vi "Begin_Turret.vi"() -> (0 "error out":errorcluster)   [LabVIEW 2012]
uses:
  <vilib>/Rock Robotics/WPI/CAN/Jaguar/SubVIs/WPI_CANJaguar_ControlMode.ctl
  <vilib>/Rock Robotics/WPI/CAN/Jaguar/SubVIs/WPI_CANJaguar_PositionReference.ctl
  <vilib>/Rock Robotics/WPI/MotorControl/WPI_MotorControlOpenCANJaguar.vi
panel:
  out "Succeeded?":bool
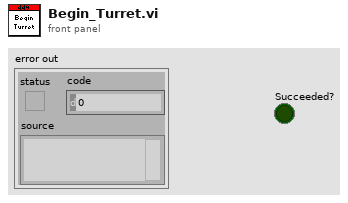
[diagram p1: front panel]
types:
  T1 = typedef "WPI_CANJaguar_ControlMode.ctl" = enum8{"Percent VBus", "Current", "Speed", "Position", "Voltage"}
  T2 = typedef "WPI_MotorControlDeviceRef.ctl" = cluster{"DeviceStatus":errorcluster, "Type":enum16{"PWM", "CAN"}, "PWM":cluster{"Digital Module":T3, "PWM Channel":T4, "DeadBand":T5}, "CAN":cluster{"Device Number":u8, "Control Mode":T1, "Semaphore":T6, "Max Vout":dbl}, "Invert":bool, "TransformRef":T7, "InvTransformRef":T7}
  T3 = typedef "FPGA_TypedefDigitalModule.ctl" = enum16{"Digital Module 1", "Digital Module 2"}
  T4 = typedef "FPGA_DIOPWMChannel.ctl" = enum8{"PWM 1", "PWM 2", "PWM 3", "PWM 4", "PWM 5", "PWM 6", "PWM 7", "PWM 8", "PWM 9", "PWM 10", "Invalid"}
  T5 = typedef "WPI_PWMDeadband.ctl" = cluster{"Name":string, "maxPositivePwm":i32, "minPositivePwm":i32, "centerPwm":i32, "maxNegativePwm":i32, "minNegativePwm":i32, "angularRange":u16}
  T6 = typedef "Semaphore RefNum" = refnum<k1>
  T7 = typedef "WPI_PWMTransform_ConPane.ctl" = refnum<vi>
  T8 = typedef "WPI_CANJaguar_PositionReference.ctl" = u8
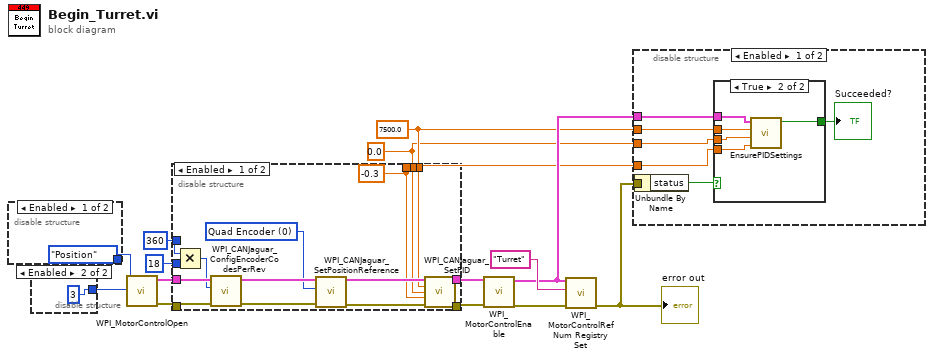
[diagram p0: block diagram]
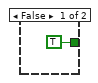
[diagram p2: hidden frame]
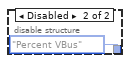
[diagram p5: hidden frame]
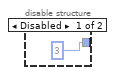
[diagram p6: hidden frame]
diagram:
  w2 = 0.0 ("P")
  w3 = 7500.0 ("P")
  n1 = disable-structure shown="Enabled" {
    disable-tunnel: [WPI_CANJaguar_ControlMode."Position" ("Control Mode") WPI_CANJaguar_ControlMode."Percent VBus" ("Control Mode")] -> w14
    frame Enabled {
    }
    frame Disabled {
    }
  }
  n2 = disable-structure shown="Enabled" {
    disable-tunnel: [u8 3 ("Device Number") u8 3 ("Device Number")] -> w15
    frame Disabled {
    }
    frame Enabled {
    }
  }
  n3 = call-poly <vilib>:"WPI_MotorControlOpen.vi"("Device Number"=w15, "Control Mode"=w14) -> ("error out"=w12:errorcluster, "MotorControlDeviceRef"=w13:T2)  [unwired: 8 in]
  n4 = disable-structure shown="Enabled" {
    disable-tunnel: w13 -> [w34 w36]
    disable-tunnel: w12 -> [w33 w35]
    disable-tunnel: [w27 w36] -> w11
    disable-tunnel: [w26 w35] -> w10
    disable-tunnel: u16 360 -> [w25 _]
    disable-tunnel: u16 18 ("y") -> [w23 _]
    disable-tunnel: w3 -> [w22 _]
    disable-tunnel: w2 -> [w21 _]
    disable-tunnel: [w20 _] -> w1
    frame Enabled {
      w20 = -0.3 ("P")
      w30 = T8 0 items=["Quad Encoder"=0, "Potentiometer"=1, "None"=255] ("Position Reference")
      n5 = Multiply(x=w25, y=w23) -> (x*y=w24:u16)
      n6 = call <vilib>:"WPI_CANJaguar_ConfigEncoderCodesPerRev.vi"("error in (no error)"=w33, "Encoder Codes Per Rev"=w24, "CAN Jaguar Ref"=w34) -> ("error out"=w32:errorcluster, "CAN Jaguar Ref Out"=w31:T2)  [unwired: 7 in]
      n7 = call <vilib>:"WPI_CANJaguar_SetPositionReference.vi"("error in (no error)"=w32, "Position Reference"=w30, "CAN Jaguar Ref"=w31) -> ("error out"=w28:errorcluster, "CAN Jaguar Ref Out"=w29:T2)  [unwired: 7 in]
      n8 = call <vilib>:"WPI_CANJaguar_SetPID.vi"("CAN Jaguar Ref"=w29, "P"=w22, "I"=w21, "D"=w20, "error in (no error)"=w28) -> ("CAN Jaguar Ref Out"=w27:T2, "error out"=w26:errorcluster)  [unwired: 9 in]
    }
    frame Disabled {
    }
  }
  n9 = call <vilib>:"WPI_MotorControlEnable.vi"("error in (no error)"=w10, "CAN Jaguar Ref"=w11) -> ("error out"=w9:errorcluster, "CAN Jaguar Ref Out"=w4:T2)  [unwired: 8 in]
  n10 = call <vilib>:"WPI_MotorControlRefNum Registry Set.vi"("error in (no error)"=w9, "refnum name"="Turret", "MotorControlDevRef"=w4) -> ("error out"=w5:errorcluster)  [unwired: 7 in, 1 out]
  "error out" <- w5
  n11 = disable-structure shown="Enabled" {
    disable-tunnel: w5 -> [w41 _]
    disable-tunnel: w4 -> [w40 _]
    disable-tunnel: w3 -> [w39 _]
    disable-tunnel: w2 -> [w38 _]
    disable-tunnel: w1 -> [w37 _]
    frame Enabled {
      n12 = Unbundle By Name(w41) -> ("status"=w43:bool)
      n13 = case shown="True" w43 {
        tunnel: w40 -> [_ w49]
        tunnel: w39 -> [_ w48]
        tunnel: w38 -> [_ w47]
        tunnel: w37 -> [_ w46]
        tunnel: [TRUE ("Succeeded?") w45] -> w42
        frame False {
        }
        frame True {
          n14 = call "EnsurePIDSettings.vi"("D"=w46, "I"=w47, "P"=w48, "CAN Jaguar Ref"=w49) -> ("Succeeded?"=w45:bool)  [unwired: 7 in]
        }
      }
      "Succeeded?" <- w42
    }
    frame Disabled {
    }
  }
